vi "SingleServiceRegistered_InvalidResolveRequests_Error.vi"() -> (6 "Pass":bool, 15 "error out":errorcluster)   [LabVIEW 2020]
uses:
  Discovery_client/RPC Messages/ni_measurementlink_discovery_v1_ServiceDescriptor.ctl
  Discovery_client/Discovery_client.lvlib
  Discovery_client/RPC Messages/ni_measurementlink_discovery_v1_ServiceLocation.ctl
  Discovery_client/RPC Messages/ni_measurementlink_discovery_v1_RegisterServiceRequest.ctl
  Discovery_client/RPC Messages/ni_measurementlink_discovery_v1_ResolveServiceRequest.ctl
panel:
  out "Empty provided_interface fails (as expected)?":bool
  out "Wrong provided_interface fails (as expected)?":bool
  out "Empty provided_interface correct service_class fails (as expected)?":bool
  out "Wrong provided_interface correct service_class fails (as expected)?":bool
  out "Correct provided_interface wrong service_class fails (as expected)?":bool
  # "Test assumes discovery service has already been started."
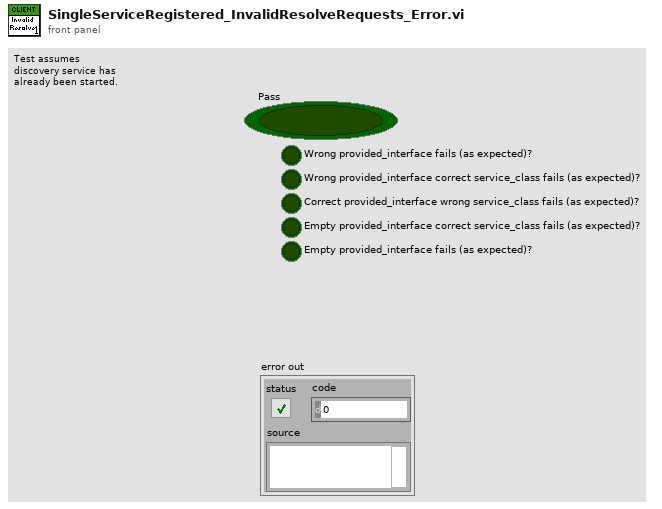
[diagram p1: front panel]
types:
  T1 = typedef "Discovery_client.lvlib/ni_measurementlink_discovery_v1_ResolveServiceRequest.ctl" = cluster{"provided_interface":string, "service_class":string}
  T2 = typedef "Discovery_client.lvlib/ni_measurementlink_discovery_v1_RegisterServiceRequest.ctl" = cluster{"service_description":T3, "location":T4}
  T3 = typedef "Discovery_client.lvlib/ni_measurementlink_discovery_v1_ServiceDescriptor.ctl" = cluster{"display_name":string, "description_url":string, "provided_interfaces":string[], "service_class":string, "attributes":string[]}
  T4 = typedef "Discovery_client.lvlib/ni_measurementlink_discovery_v1_ServiceLocation.ctl" = cluster{"location":string, "insecure_port":string, "ssl_authenticated_port":string}
  T5 = typedef "Discovery_client.lvlib/ni_measurementlink_discovery_v1_RegisterServiceResponse.ctl" = cluster{"registration_id":string}
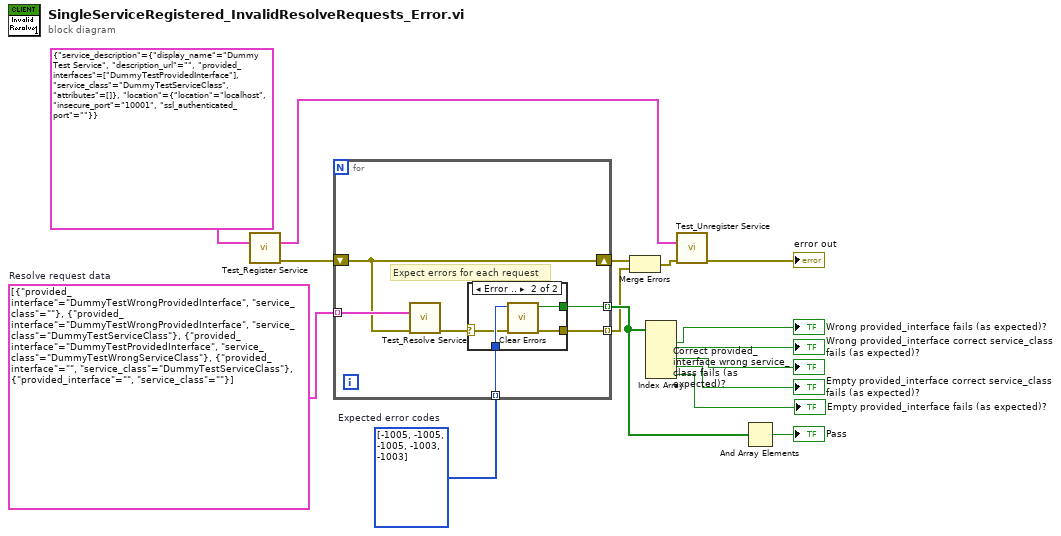
[diagram p0: block diagram]
diagram:
  w4 = i32[] [-1005, -1005, -1005, -1003, -1003]  # Expected error codes
  w12 = T1[] [{"provided_interface"="DummyTestWrongProvidedInterface", "service_class"=""}, {"provided_interface"="DummyTestWrongProvidedInterface", "service_class"="DummyTestServiceClass"}, {"provided_interface"="DummyTestProvidedInterface", "service_class"="DummyTestWrongServiceClass"}, {"provided_interface"="", "service_class"="DummyTestServiceClass"}, {"provided_interface"="", "service_class"=""}]  # Resolve request data
  n1 = call "Test_Register Service.vi"("Request Data"=T2 {"service_description"={"display_name"="Dummy Test Service", "description_url"="", "provided_interfaces"=["DummyTestProvidedInterface"], "service_class"="DummyTestServiceClass", "attributes"=[]}, "location"={"location"="localhost", "insecure_port"="10001", "ssl_authenticated_port"=""}}) -> ("Response Data"=w16:T5, "error out"=w14:errorcluster)  [unwired: 13 in]
  n2 = for {
    tunnel: w12 -> [w22] mode=indexing
    shift-right: [w21] -> w3
    shift-left: w14 -> [w21]
    tunnel: [w17] -> w6 mode=indexing
    tunnel: w4 -> [w19] mode=indexing
    tunnel: [w18] -> w1 mode=indexing
    # "Expect errors for each request"
    n3 = call "Test_Resolve Service.vi"("Request Data"=w22, "error in (no error)"=w21) -> ("error out"=w20:errorcluster)  [unwired: 12 in, 1 out]
    n4 = case shown="Error .." w20 {
      selector: w20 -> [w23 w24]
      tunnel: [_ w27] -> w17
      tunnel: [w23 w26] -> w18
      tunnel: w19 -> [_ w25]
      frame No Error {
      }
      frame Error {
        n5 = call <vilib>:"Clear Errors.vi"("error in (no error)"=w24, "specific error code to clear (0: all)"=w25) -> ("error out"=w26:errorcluster, "specific error cleared?"=w27:bool)  [unwired: 4 in]
      }
    }
  }
  n6 = Merge Errors(w3, w1) -> (w2:errorcluster)
  n7 = Index Array(array=w6) -> (element #1=→"Wrong provided_interface fails (as expected)?":bool, element #2=→"Wrong provided_interface correct service_class fails (as expected)?":bool, element #3=→"Correct provided_interface wrong service_class fails (as expected)?":bool, element #4=→"Empty provided_interface correct service_class fails (as expected)?":bool, element #5=→"Empty provided_interface fails (as expected)?":bool)  [unwired: 5 in]
  n8 = call "Test_Unregister Service.vi"("Request Data"=w16, "error in (no error)"=w2) -> ("error out"=→"error out":errorcluster)  [unwired: 12 in, 1 out]
  n9 = And Array Elements(Boolean array=w6) -> (logical AND=→"Pass":bool)
